vi "Convert AcquireParams to Array.vi"(1 "ACQUIPARAMS":T1 {"CFA"."CFA" items=["CFA_NONE", "CFA_VRI", "CFA_VRIV6", "CFA_BAYER", "CFA_BAYERFLIP"]; "TriggerTime"."fractions" format="%32.0f"}) -> (0 "ACQUIPARAMS Data Array":u32[](array[numeric]))   [LabVIEW 2013, in "VRI.lvlib"]
uses:
  VRI.lvlib
  _Type Defs/PHCon ACQUIPARAMS.ctl
  _Type Defs/PhCon SyncImaging.ctl
  _Type Defs/Rect.ctl
  _Type Defs/PHCon Time64.ctl
  _Type Defs/PhInt CFA.ctl
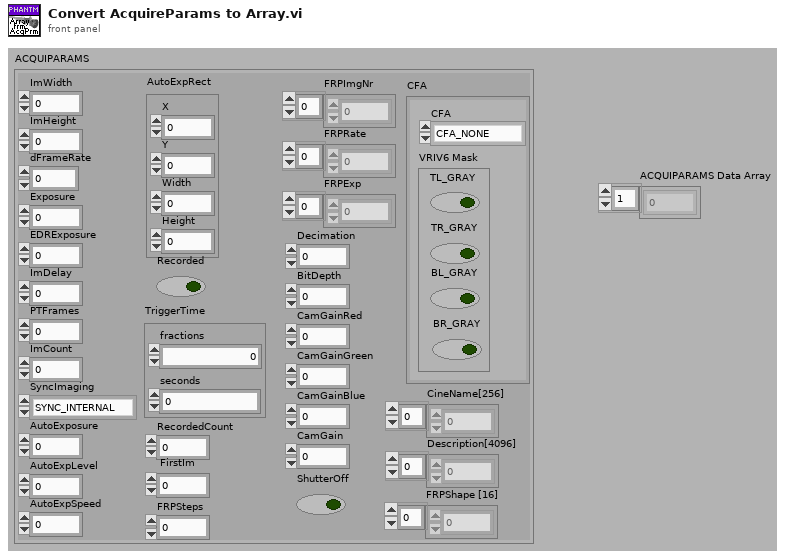
[diagram p1: front panel]
types:
  T1 = typedef "VRI.lvlib/PHCon ACQUIPARAMS.ctl" = cluster{"ImWidth":u32, "ImHeight":u32, "(deprecated)FrameRateInt":u32, "Exposure":u32, "EDRExposure":u32, "ImDelay":u32, "PTFrames":u32, "ImCount":u32, "SyncImaging":T2, "AutoExposure":u32, "AutoExpLevel":u32, "AutoExpSpeed":u32, "AutoExpRect":T3, "Recorded":bool, "TriggerTime":T4, "RecordedCount":u32, "FirstIm":i32, "FRPSteps":u32, "FRPImgNr":i32[], "FRPRate":u32[], "FRPExp":u32[], "Decimation":u32, "BitDepth":u32, "CamGainRed":u32, "CamGainGreen":u32, "CamGainBlue":u32, "CamGain":u32, "ShutterOff":bool, "CFA":T5, "CineName[256]":u8[], "Description[4096]":u8[], "FRPShape [16]":u32[], "dFrameRate":dbl}
  T2 = typedef "VRI.lvlib/PhCon SyncImaging.ctl" = enum32{"SYNC_INTERNAL", "SYNC_EXTERNAL", "SYNC_LOCKTOIRIG"}
  T3 = typedef "VRI.lvlib/Rect.ctl" = cluster{"X":i32, "Y":i32, "Width":i32, "Height":i32}
  T4 = typedef "VRI.lvlib/PHCon Time64.ctl" = cluster{"fractions":u32, "seconds":u32}
  T5 = typedef "VRI.lvlib/PhInt CFA.ctl" = cluster{"CFA":u32, "VRIV6 Mask":cluster{"TL_GRAY":bool, "TR_GRAY":bool, "BL_GRAY":bool, "BR_GRAY":bool}}
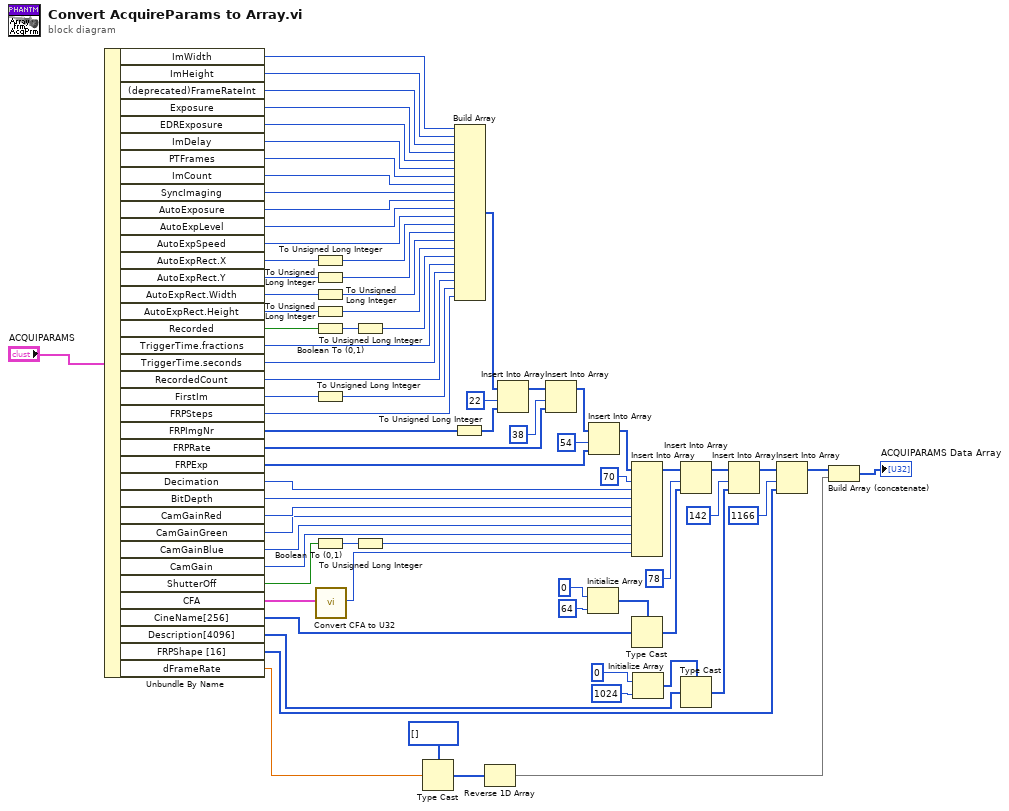
[diagram p0: block diagram]
diagram:
  n1 = Unbundle By Name("ACQUIPARAMS") -> ("ImWidth"=w52:u32, "ImHeight"=w53:u32, "(deprecated)FrameRateInt"=w54:u32, "Exposure"=w55:u32, "EDRExposure"=w56:u32, "ImDelay"=w57:u32, "PTFrames"=w58:u32, "ImCount"=w59:u32, "SyncImaging"=w60:T2, "AutoExposure"=w61:u32, "AutoExpLevel"=w62:u32, "AutoExpSpeed"=w63:u32, "AutoExpRect.X"=w68:i32, "AutoExpRect.Y"=w69:i32, "AutoExpRect.Width"=w70:i32, "AutoExpRect.Height"=w71:i32, "Recorded"=w49:bool, "TriggerTime.fractions"=w50:u32, "TriggerTime.seconds"=w72:u32, "RecordedCount"=w73:u32, "FirstIm"=w74:i32, "FRPSteps"=w75:u32, "FRPImgNr"=w46:i32[], "FRPRate"=w42:u32[], "FRPExp"=w39:u32[], "Decimation"=w36:u32, "BitDepth"=w35:u32, "CamGainRed"=w34:u32, "CamGainGreen"=w33:u32, "CamGainBlue"=w32:u32, "CamGain"=w31:u32, "ShutterOff"=w29:bool, "CFA"=w27:T5, "CineName[256]"=w22:u8[], "Description[4096]"=w18:u8[], "FRPShape [16]"=w10:u32[], "dFrameRate"=w7:dbl)
  n2 = To Unsigned Long Integer(number=w68) -> (unsigned 32bit integer=w64:u32)
  n3 = To Unsigned Long Integer(number=w69) -> (unsigned 32bit integer=w66:u32)
  n4 = To Unsigned Long Integer(number=w70) -> (unsigned 32bit integer=w65:u32)
  n5 = To Unsigned Long Integer(number=w71) -> (unsigned 32bit integer=w67:u32)
  n6 = Boolean To (0,1)(Boolean=w49) -> (0, 1=w48:i16)
  n7 = To Unsigned Long Integer(number=w74) -> (unsigned 32bit integer=w76:u32)
  n8 = Boolean To (0,1)(Boolean=w29) -> (0, 1=w30:i16)
  n9 = call "Convert CFA to U32.vi"("CFA in"=w27) -> ("CFA out"=w26:u32)  [unwired: 18 out]
  n10 = To Unsigned Long Integer(number=w48) -> (unsigned 32bit integer=w47:u32)
  n11 = To Unsigned Long Integer(number=w30) -> (unsigned 32bit integer=w28:u32)
  n12 = Type Cast(type=u32[] [], x=w7) -> (*(type *) &x=w1:u32[])
  n13 = To Unsigned Long Integer(number=w46) -> (unsigned 32bit integer=w45:u32[])
  n14 = Build Array(w52, w53, w54, w55, w56, w57, w58, w59, w60, w61, w62, w63, w64, w66, w65, w67, w47, w50, w72, w73, w76, w75) -> (w6:u32[])
  n15 = Reverse 1D Array(array=w1) -> (reversed array=w3:u32[])
  n16 = Insert Into Array(array=w6, index=22, new element=w45) -> (w5:u32[])
  n17 = Insert Into Array(array=w5, index=38, new element=w42) -> (w40:u32[])
  n18 = Initialize Array(u32 0 ("element"), 64 ("dimension size")) -> (w25:u32[])
  n19 = Insert Into Array(array=w40, index=54, new element=w39) -> (w38:u32[])
  n20 = Insert Into Array(array=w38, index=70, new element #1=w36, new element #2=w35, new element #3=w34, new element #4=w33, new element #5=w32, new element #6=w31, new element #7=w28, new element #8=w26) -> (w17:u32[])
  n21 = Type Cast(type=w25, x=w22) -> (*(type *) &x=w15:u32[])
  n22 = Initialize Array(u32 0 ("element"), 1024 ("dimension size")) -> (w21:u32[])
  n23 = Insert Into Array(array=w17, index=78, new element=w15) -> (w14:u32[])
  n24 = Type Cast(type=w21, x=w18) -> (*(type *) &x=w13:u32[])
  n25 = Insert Into Array(array=w14, index=142, new element=w13) -> (w11:u32[])
  n26 = Insert Into Array(array=w11, index=1166, new element=w10) -> (w8:u32[])
  n27 = Build Array (concatenate)(w8, w3) -> (→"ACQUIPARAMS Data Array":u32[])
